vi "XY muliti ch chart.vi"(6 "lenth":i32=1000, 8 "clear?":bool, 10 "Data":dbl[](array[numeric]), 11 "current time":timestamp) -> (2 "XY Graph":cluster{cluster{"time":dbl, "Y":dbl}[]}[](graph))   [LabVIEW 2011]
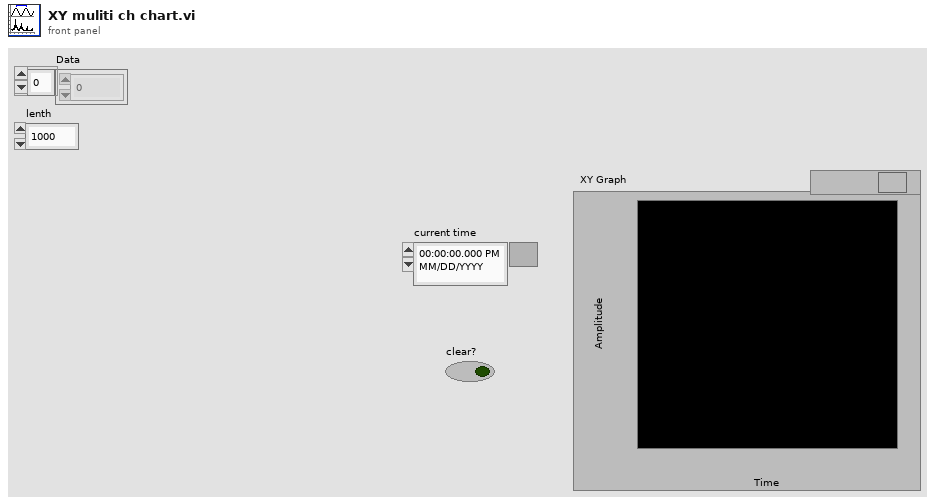
[diagram p1: front panel]
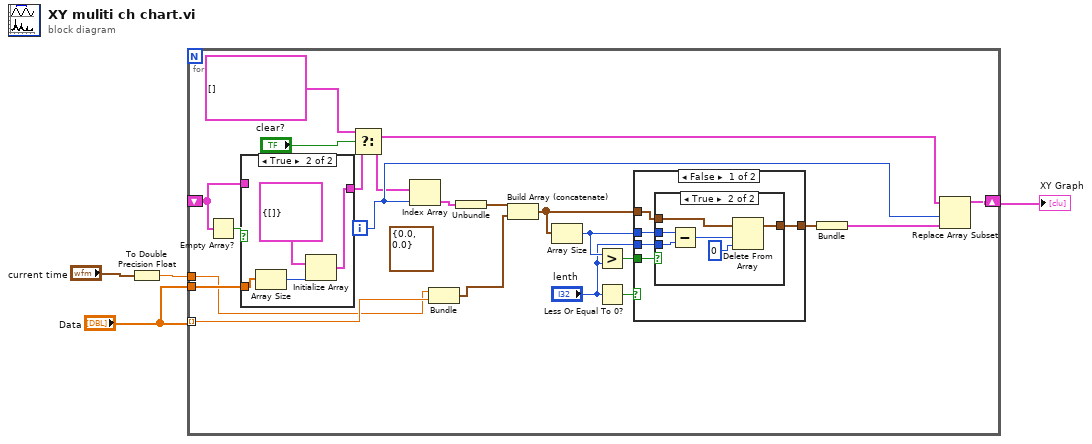
[diagram p0: block diagram]
diagram:
  n1 = To Double Precision Float(number="current time") -> (double precision float=w3:dbl)
  n2 = for {
    tunnel: "Data" -> [w6] mode=indexing
    tunnel: w3 -> [w5]
    shift-right: [w22] -> w2
    shift-left: _ -> [w9]
    tunnel: "Data" -> [w10]
    i -> [w23]
    (unwired) cluster{"time":dbl, "Y":dbl} {"time"=0.0, "Y"=0.0} ("cluster")
    n3 = Empty Array?(array=w9) -> (empty?=w11:bool)
    n4 = case shown="True" w11 {
      tunnel: w10 -> [_ w29]
      tunnel: [w26 w27] -> w8
      tunnel: w9 -> [w26 _]
      frame False {
      }
      frame True {
        n5 = Array Size(array=w29) -> (size(s)=w28:i32)
        n6 = Initialize Array(cluster{cluster{"time":dbl, "Y":dbl}[]} {[]}, w28) -> (w27:cluster{cluster{"time":dbl, "Y":dbl}[]}[])
      }
    }
    n7 = Select(t=cluster{cluster{"time":dbl, "Y":dbl}[]}[] [] ("array of clusters"), s="clear?", f=w8) -> (s? t:f=w21:cluster{cluster{"time":dbl, "Y":dbl}[]}[])
    n8 = Index Array(array=w21, index=w23) -> (element=w25:cluster{cluster{"time":dbl, "Y":dbl}[]})
    n9 = Bundle(w5, w6) -> (w7:cluster{dbl, dbl})  [unwired: 1 in]
    n10 = Unbundle(w25) -> (w24:cluster{"time":dbl, "Y":dbl}[])
    n11 = Build Array (concatenate)(w24, w7) -> (w18:cluster{"time":dbl, "Y":dbl}[])
    n12 = Array Size(array=w18) -> (size(s)=w17:i32)
    n13 = Greater?(x=w17, y="lenth") -> (0:w14:bool)
    n14 = Less Or Equal To 0?(x="lenth") -> (x <= 0?=w12:bool)
    n15 = case shown="False" w12 {
      tunnel: w18 -> [w35 w43]
      tunnel: w17 -> [w34 _]
      tunnel: [w33 w43] -> w15
      tunnel: w14 -> [w32 _]
      tunnel: "lenth" -> [w31 _]
      frame False {
        n16 = case shown="True" w32 {
          tunnel: w35 -> [w36 w42]
          tunnel: w34 -> [_ w40]
          tunnel: w31 -> [_ w39]
          tunnel: [w36 w37] -> w33
          frame False {
          }
          frame True {
            n17 = Subtract(x=w40, y=w39) -> (x-y=w38:i32)
            n18 = Delete From Array(array=w42, length=w38, index=0) -> (array with subset deleted=w37:cluster{"time":dbl, "Y":dbl}[])  [unwired: 1 out]
          }
        }
      }
      frame True {
      }
    }
    n19 = Bundle(w15) -> (w16:cluster{cluster{"time":dbl, "Y":dbl}[]})  [unwired: 1 in]
    n20 = Replace Array Subset(array=w21, new element=w16, index=w23) -> (w22:cluster{cluster{"time":dbl, "Y":dbl}[]}[])
  }
  "XY Graph" <- w2
